vi "Limits(Switch+Encoder).vi"(4 "Into Home Limit Is Pos (Encoder)":bool, 6 "Into Home Limit Is Pos (Motor)":bool, 8 "Power In":dbl format="%#_13g", 9 "Encoder Limit":dbl format="%#_13g", 10 "Motor Ref":T4={"DeviceStatus"={"status"=FALSE, "code"=0, "source"=""}, "Type"=enum."PWM", "PWM"={"PWM Channel"=enum."Invalid", "DeadBand"={"Name"="", "maxPositivePwm"=0, "minPositivePwm"=0, "centerPwm"=0, "maxNegativePwm"=0, "minNegativePwm"=0, "angularRange"=0}}, "CAN"={"Device Number"=0, "SetOutput VI Ref"=variant, "GetOutput VI Ref"=variant, "Enable VI Ref"=variant, "Disable VI Ref"=variant, "Data"=variant}, "Invert"=FALSE, "DIO PWM"={"PWM \"Enable\" Channel"=enum."Invalid", "DIOChannel"=enum."Invalid", "PWM Rate"=0.0}}, 11 "Limit Switch Ref":T1={"DevStatus"={"status"=FALSE, "code"=0, "source"=""}, "DIO Channel"=enum."DIO 1", "CntIndex"=enum."Invalid", "Normally Closed"=FALSE}) -> (0 "Power Out":dbl)   [LabVIEW 2018]
uses:
  <vilib>/Rock Robotics/WPI/MotorControl/WPI_MotorControlDeviceRef.ctl
  <vilib>/Rock Robotics/WPI/MotorControl/WPI_MotorControlType.ctl
  <vilib>/Rock Robotics/SystemInterfaces/DIO/FPGA_DIOPWMChannel.ctl
  <vilib>/Rock Robotics/WPI/PWM/WPI_PWMDeadband.ctl
  <vilib>/Rock Robotics/SystemInterfaces/DIO/FPGA_DIOChannel.ctl
  <vilib>/Rock Robotics/WPI/Switch/WPI_SwitchDevRef.ctl
  <vilib>/Rock Robotics/SystemInterfaces/Counter/FPGA_CounterCtrSystemIndex.ctl
  <vilib>/Rock Robotics/WPI/ThirdParty/Phoenix-LabVIEW/Motor Controller/Get/CTRE_Phoenix_MotorController_GetSelectedSensorData.vi
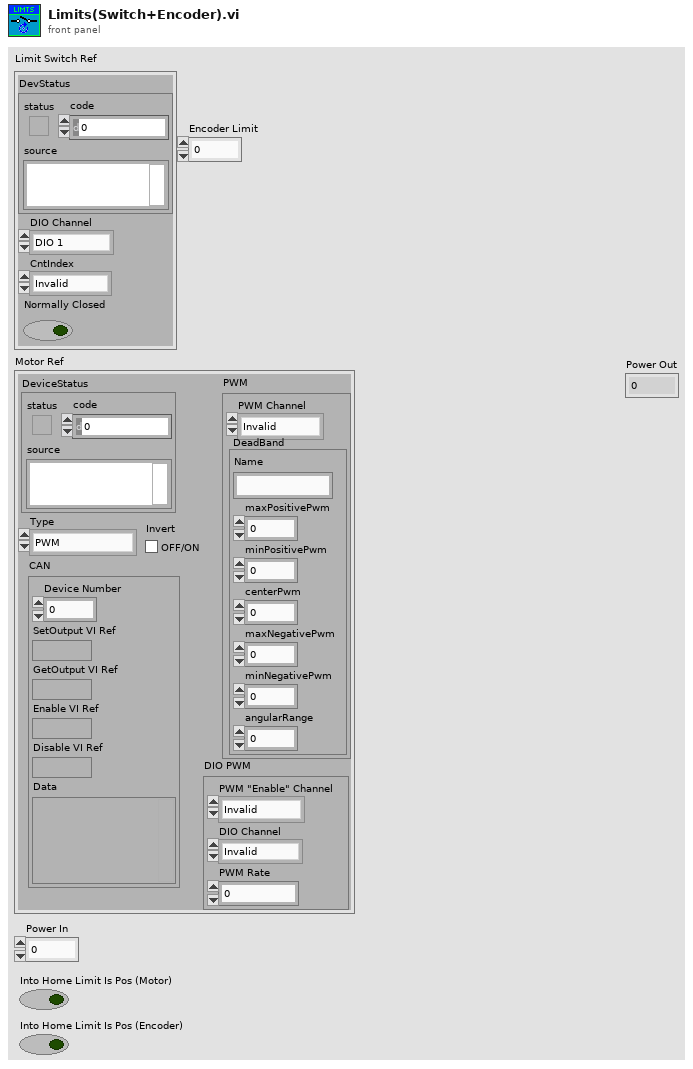
[diagram p1: front panel]
types:
  T1 = typedef "WPI_SwitchDevRef.ctl" = cluster{"DevStatus":errorcluster, "DIO Channel":T2, "CntIndex":T3, "Normally Closed":bool}
  T2 = typedef "FPGA_DIOChannel.ctl" = enum8{"DIO 0", "DIO 1", "DIO 2", "DIO 3", "DIO 4", "DIO 5", "DIO 6", "DIO 7", "DIO 8", "DIO 9", "DIO MXP 0", "DIO MXP 1", "DIO MXP 2", "DIO MXP 3", "DIO MXP 4", "DIO MXP 5", "DIO MXP 6", "DIO MXP 7", "DIO MXP 8", "DIO MXP 9", "DIO MXP 10", "DIO MXP 11", "DIO MXP 12", "DIO MXP 13", "DIO MXP 14", "DIO MXP 15", "SPI Port CS1", "SPI Port CS2", "SPI Port CS3", "SPI Port MISO", "SPI Port MOSI", "Invalid"}
  T3 = typedef "FPGA_CounterCtrSystemIndex.ctl" = enum8{"Ctr 0", "Ctr 1", "Ctr 2", "Ctr 3", "Ctr 4", "Ctr 5", "Ctr 6", "Ctr 7", "Invalid"}
  T4 = typedef "WPI_MotorControlDeviceRef.ctl" = cluster{"DeviceStatus":errorcluster, "Type":T5, "PWM":cluster{"PWM Channel":T6, "DeadBand":T7}, "CAN":cluster{"Device Number":u8, "SetOutput VI Ref":variant, "GetOutput VI Ref":variant, "Enable VI Ref":variant, "Disable VI Ref":variant, "Data":variant}, "Invert":bool, "DIO PWM":cluster{"PWM \"Enable\" Channel":T6, "DIOChannel":T2, "PWM Rate":dbl}}
  T5 = typedef "WPI_MotorControlType.ctl" = enum16{"PWM", "CAN", "DIO PWM"}
  T6 = typedef "FPGA_DIOPWMChannel.ctl" = enum8{"PWM 0", "PWM 1", "PWM 2", "PWM 3", "PWM 4", "PWM 5", "PWM 6", "PWM 7", "PWM 8", "PWM 9", "PWM MXP 0", "PWM MXP 1", "PWM MXP 2", "PWM MXP 3", "PWM MXP 4", "PWM MXP 5", "PWM MXP 6", "PWM MXP 7", "PWM MXP 8", "PWM MXP 9", "Invalid"}
  T7 = typedef "WPI_PWMDeadband.ctl" = cluster{"Name":string, "maxPositivePwm":i32, "minPositivePwm":i32, "centerPwm":i32, "maxNegativePwm":i32, "minNegativePwm":i32, "angularRange":u16}
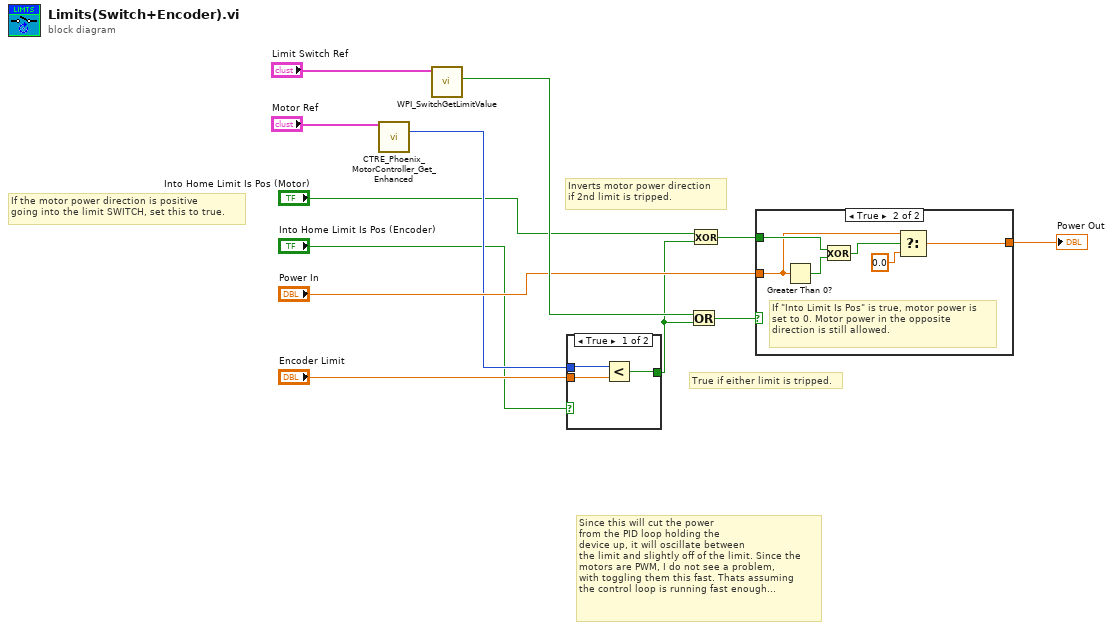
[diagram p0: block diagram]
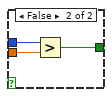
[diagram p2: hidden frame]
diagram:
  # "True if either limit is tripped."
  # "Inverts motor power direction\nif 2nd limit is tripped."
  # "Since this will cut the power\nfrom the PID loop holding the\ndevice up, it will oscillate between\nthe limit and slightly off of the limit. Since the\nmotors are PWM, I do not see a problem,\nwith toggling them this fast. Thats assuming\nthe control loop is running fast enough..."
  # "If the motor power direction is positive\ngoing into the limit SWITCH, set this to true."
  n1 = call-poly <vilib>:"CTRE_Phoenix_MotorController_Get_Enhanced.vi"("PhoenixMotorControlDevRef"="Motor Ref") -> ("Position (Raw Sensor Units)"=w6:i32)  [unwired: 11 in, 3 out]
  n2 = call <vilib>:"WPI_SwitchGetLimitValue.vi"("SwitchDevRef"="Limit Switch Ref") -> ("Switch Pressed"=w12:bool)  [unwired: 8 in, 2 out]
  n3 = case shown="True" "Into Home Limit Is Pos (Encoder)" {
    tunnel: "Encoder Limit" -> [w13 w18]
    tunnel: w6 -> [w14 w17]
    tunnel: [w15 w16] -> w3
    frame True {
      n4 = Less?(x=w14, y=w13) -> (x < y?=w15:bool)
    }
    frame False {
      n5 = Greater?(x=w17, y=w18) -> (0:w16:bool)
    }
  }
  n6 = Or(x=w12, y=w3) -> (x .or. y?=w5:bool)
  n7 = Exclusive Or(1:w3, 2:"Into Home Limit Is Pos (Motor)") -> (0:w4:bool)
  n8 = case shown="True" w5 {
    tunnel: [w19 w22] -> w10
    tunnel: w4 -> [_ w21]
    tunnel: "Power In" -> [w19 w20]
    frame False {
    }
    frame True {
      # "If \"Into Limit Is Pos\" is true, motor power is set to 0. Motor power in the opposite direction is still allowed."
      n9 = Greater Than 0?(x=w20) -> (x > 0?=w24:bool)
      n10 = Exclusive Or(1:w24, 2:w21) -> (0:w23:bool)
      n11 = Select(t=w20, s=w23, f=0.0) -> (s? t:f=w22:dbl)
    }
  }
  "Power Out" <- w10
